vi "Velmex cfg motor speed.vi"(8 "error in (no error)":errorcluster {"code" format="%.0x"}, 9 "Simulation":T1, 10 "Channel parsed command info":T2, 11 "input cluster":refnum<class "VelmexStage.lvclass">) -> (0 "error out":errorcluster, 2 "new commands":string, 3 "output cluster":refnum<class "VelmexStage.lvclass">)   [LabVIEW 2020, in "VelmexStage.lvclass"]
uses:
  VelmexStage.lvclass
  channel parsed cmd cluster.ctl
  OnOffTypeDef.ctl
  VelmexStage.lvclass/VelmexStage.ctl
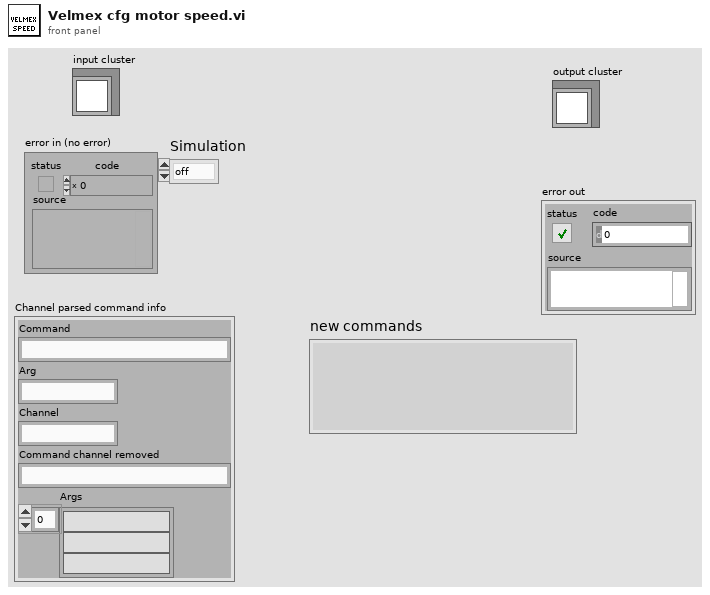
[diagram p1: front panel]
types:
  T1 = typedef "OnOffTypeDef.ctl" = enum16{"off", "on"}
  T2 = typedef "channel parsed cmd cluster.ctl" = cluster{"Command":string, "Arg":string, "Channel":string, "Command channel removed":string, "Args":string[]}
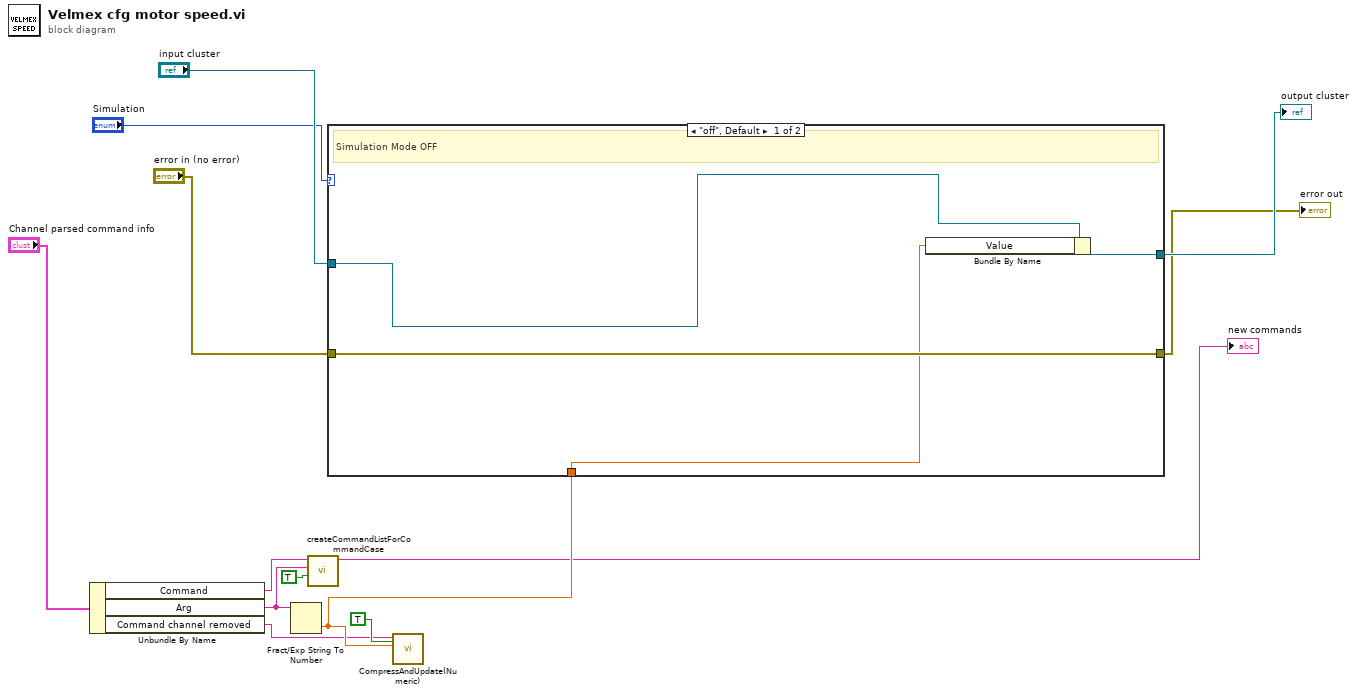
[diagram p0: block diagram]
diagram:
  n1 = Unbundle By Name("Channel parsed command info") -> ("Command"=w11:string, "Arg"=w13:string, "Command channel removed"=w1:string)
  n2 = Fract/Exp String To Number(string=w13) -> (number=w9:dbl)  [unwired: 3 in, 1 out]
  n3 = call "createCommandListForCommandCase.vi"("immediate Check (only once)"=TRUE, "setvalue"=w13, "command"=w11) -> ("new commands"=→"new commands":string)  [unwired: 8 in]
  n4 = case shown="\"off\", Default" "Simulation" {
    tunnel: [w15 w18] -> w5
    tunnel: w9 -> [w14 _]
    tunnel: "input cluster" -> [w17 w19]
    tunnel: "error in (no error)" -> [w15 w18]
    tunnel: [w16 w19] -> w6
    frame "off", Default {
      # "Simulation Mode OFF"
      n5 = Bundle By Name(cluster=w17, "Value"=w14) -> (w16:refnum<class "VelmexStage.lvclass">)
    }
    frame "on" {
      # "Simulation Mode ON"
    }
  }
  "output cluster" <- w6
  "error out" <- w5
  n6 = call "CompressAndUpdate(Numeric).vi"("force CVT update (false)"=TRUE ("force CVT update"), "Numeric"=w9, "command or variable name"=w1) -> ()  [unwired: 8 in, 1 out]
